vi "Log In.vi"(8 "error in (no error)":errorcluster, 10 "element":string, 11 "Master in":refnum<class "MASTER.lvclass">) -> (0 "error out":errorcluster, 2 "x >= 0?":bool, 3 "Master out":refnum<class "MASTER.lvclass">)   [LabVIEW 2014, in "Files Library.lvlib" / "Master.lvclass"]
uses:
  MASTER/MASTER.lvclass
  MASTER/MASTER.lvclass/MASTER.ctl
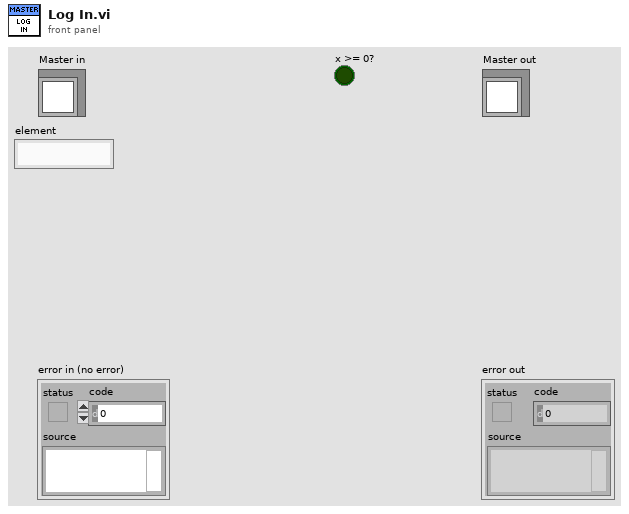
[diagram p1: front panel]
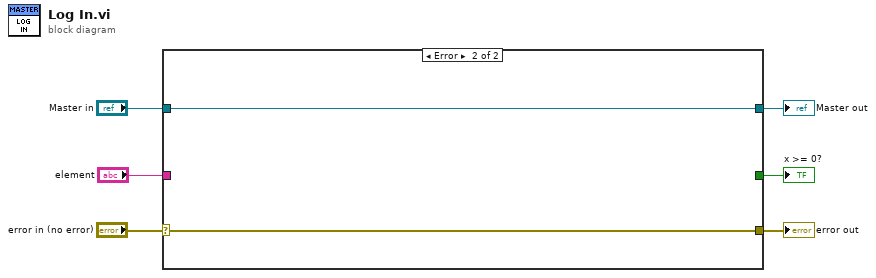
[diagram p0: block diagram]
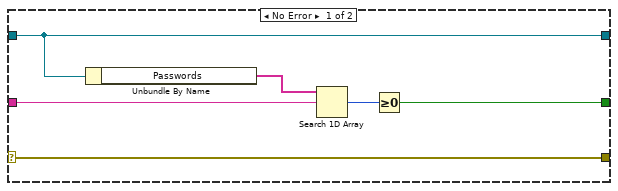
[diagram p2: hidden frame]
diagram:
  n1 = case shown="Error" "error in (no error)" {
    selector: "error in (no error)" -> [w12 w14]
    tunnel: [w12 w14] -> w5
    tunnel: [w11 w13] -> w3
    tunnel: "Master in" -> [w11 w13]
    tunnel: "element" -> [w9 _]
    tunnel: [w7 _] -> w1
    frame No Error {
      n2 = Unbundle By Name(w11) -> ("Passwords"=w10:string[])
      n3 = Search 1D Array(1D array=w10, element=w9) -> (index of element=w8:i32)  [unwired: 1 in]
      n4 = Greater Or Equal To 0?(x=w8) -> (x >= 0?=w7:bool)
    }
    frame Error {
    }
  }
  "error out" <- w5
  "Master out" <- w3
  "x >= 0?" <- w1
